vi "HasCommandArray_Query.vi"(0 "System no.":i32=1 min=1 max=4 step=1, 1 "Command":string[](array[string]), 3 "Check HLP?":bool, 4 "HLP? answer":string, 5 "error in":errorcluster) -> (14 "Available GCS commands":string[](array[string]), 15 "Is command available?":bool[](array[boolean]), 19 "error out":errorcluster)   [LabVIEW 2020]
doc: "Polymorphic VI instance for Is command present in HLP? answer.vi.\nThis VI checks whether the specified commands are present in the HLP? answer.\n\nIf Check HLP? is TRUE, HLP?.vi will be called to get HLP? information.\nIf Check HLP? is FALSE, a valid HLP? answer has to be provided in HLP answer."
panel:
  # "Is Command present in HLP answer?.vi\n\nThis VI checks whether the specified commands are present in the HLP? answer.\n\nIf \"Check HLP?\" is TRUE, HLP?.vi will be called to get HLP? information.\nIf \"Check HLP?\" is FALSE, a valid HLP? answer has to be provided in \"HLP answer\"."
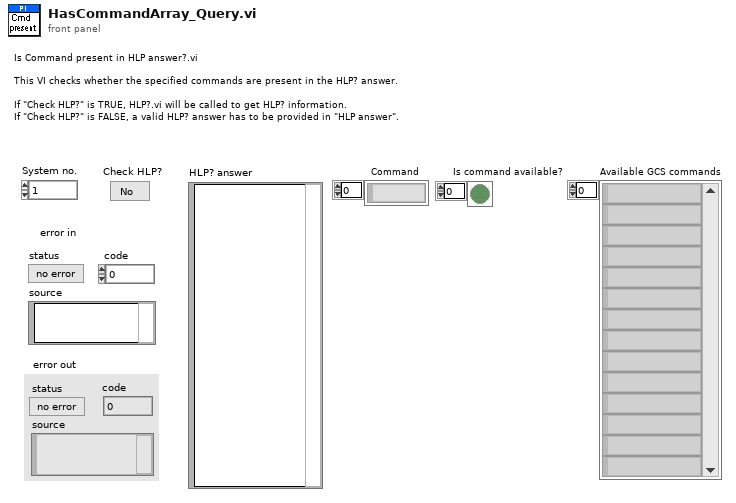
[diagram p1: front panel]
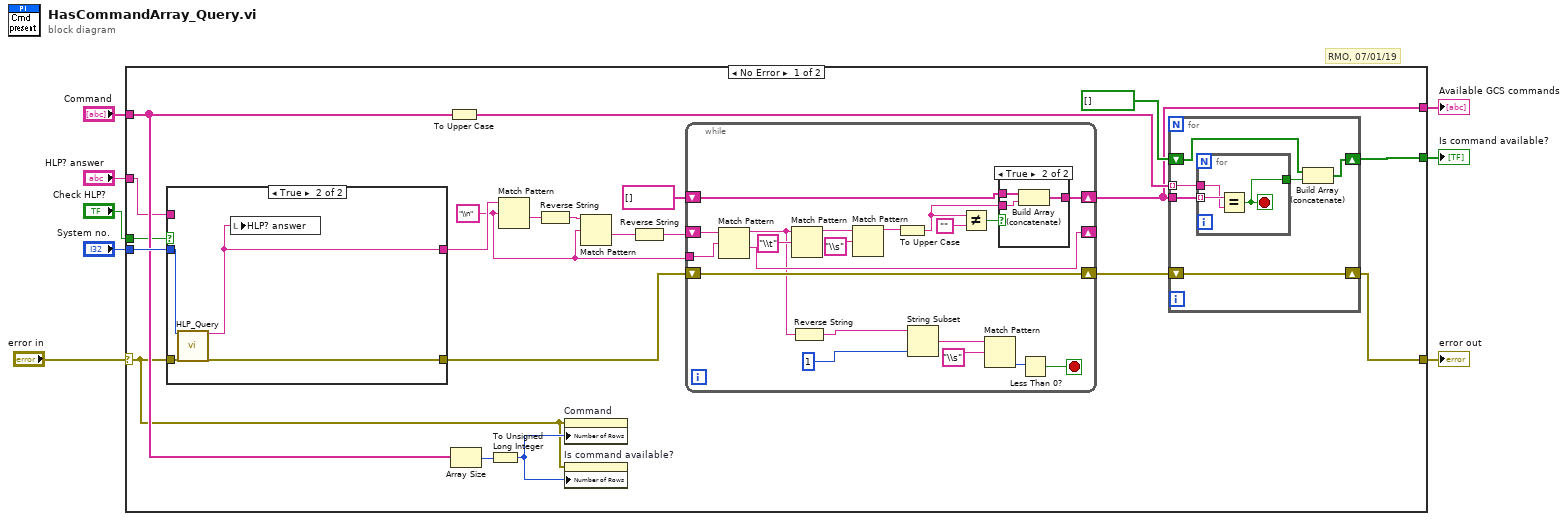
[diagram p0: block diagram]
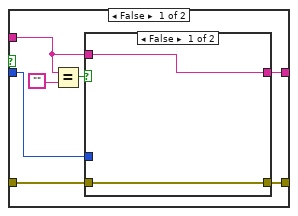
[diagram p2: hidden frame]
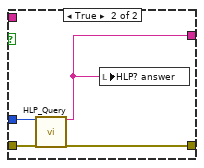
[diagram p3: hidden frame]
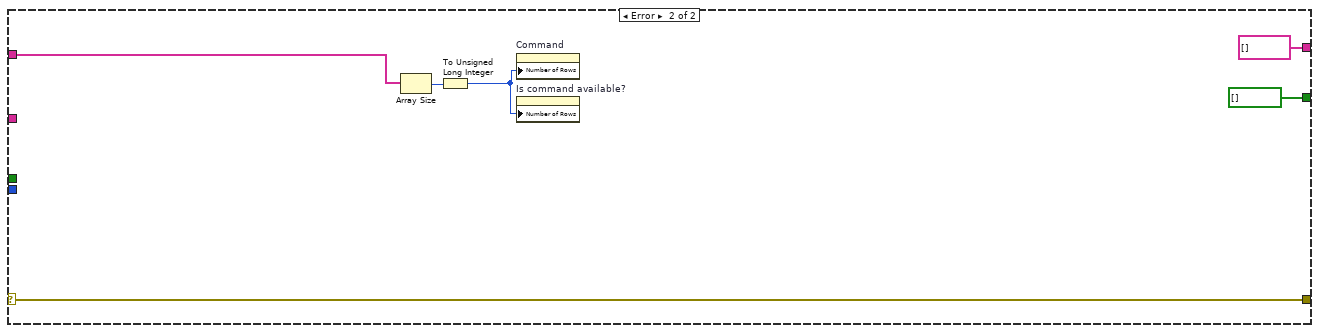
[diagram p5: hidden frame]
diagram:
  # "RMO, 07/01/19"
  n1 = case shown="No Error" "error in" {
    selector: "error in" -> [w9 w80]
    tunnel: [w23 w80] -> w8
    tunnel: "System no." -> [w29 _]
    tunnel: "Command" -> [w14 w82]
    tunnel: [w22 string[] []] -> w5
    tunnel: [w21 bool[] []] -> w4
    tunnel: "Check HLP?" -> [w11 _]
    tunnel: "HLP? answer" -> [w10 _]
    frame No Error {
      w17 = "\\n" ("regular expression")
      n2 = case shown="True" w11 {
        tunnel: w29 -> [w32 w46]
        tunnel: [w30 w43] -> w20
        tunnel: [w33 w45] -> w15
        tunnel: w9 -> [w34 w44]
        tunnel: w10 -> [w31 _]
        frame False {
          n3 = Equal?(x=w31, y="") -> (x = y?=w35:bool)
          n4 = case shown="False" w35 {
            tunnel: w34 -> [w38 w42]
            tunnel: [w38 w41] -> w33
            tunnel: w32 -> [_ w40]
            tunnel: w31 -> [w37 _]
            tunnel: [w37 w39] -> w30
            frame False {
            }
            frame True {
              n5 = call "HLP_Query.vi"("System no."=w40, "error in"=w42) -> ("Help string"=w39:string, "error out"=w41:errorcluster)  [unwired: 16 out]
              n6 = local write "HLP? answer"(w39) -> ()
            }
          }
        }
        frame True {
          n7 = call "HLP_Query.vi"("System no."=w46, "error in"=w44) -> ("Help string"=w43:string, "error out"=w45:errorcluster)  [unwired: 16 out]
          n8 = local write "HLP? answer"(w43) -> ()
        }
      }
      n9 = To Upper Case(1:w14) -> (0:w26:string[])
      n10 = Array Size(array=w14) -> (size(s)=w13:i32)
      n11 = To Unsigned Long Integer(number=w13) -> (unsigned 32bit integer=w12:u32)
      n12 = Match Pattern(string=w20, regular expression=w17) -> (after substring=w19:string)  [unwired: 4 out]
      n13 = Reverse String(1:w19) -> (0:w18:string)
      n14 = property on="Command" class="Arr (strict)"(error in=w9, "Number of Rows"=w12) -> ()  [unwired: 1 in, 2 out]
      n15 = property on="Is command available?" class="Arr (strict)"(error in=w9, "Number of Rows"=w12) -> ()  [unwired: 1 in, 2 out]
      n16 = Match Pattern(string=w18, regular expression=w17) -> (after substring=w16:string)  [unwired: 4 out]
      n17 = Reverse String(1:w16) -> (0:w28:string)
      n18 = while {
        tunnel: w17 -> [w69]
        shift-right: [w65] -> _
        shift-left: w28 -> [w68]
        shift-right: [w73] -> w22
        shift-left: string[] [] -> [w74]
        shift-right: [w67] -> w24
        shift-left: w15 -> [w67]
        stop <- w75 stop-if-true
        n19 = Match Pattern(string=w68, regular expression=w69) -> (before substring=w63:string, after substring=w65:string)  [unwired: 3 out]
        n20 = Match Pattern(string=w63, regular expression="\\t") -> (before substring=w58:string)  [unwired: 4 out]
        n21 = Reverse String(1:w63) -> (0:w62:string)
        n22 = Match Pattern(string=w58, regular expression="\\s") -> (before substring=w56:string)  [unwired: 4 out]
        n23 = To Upper Case(1:w56) -> (0:w72:string)
        n24 = String Subset(string=w62, length (rest)=1) -> (substring=w60:string)  [unwired: 1 out]
        n25 = Not Equal?(x=w72, y="") -> (x != y?=w70:bool)
        n26 = Match Pattern(string=w60, regular expression="\\s") -> (offset past match=w64:i32)  [unwired: 4 out]
        n27 = case shown="True" w70 {
          tunnel: w74 -> [w76 w79]
          tunnel: [w76 w78] -> w73
          tunnel: w72 -> [_ w77]
          frame False {
          }
          frame True {
            n28 = Build Array (concatenate)(w79, w77) -> (w78:string[])
          }
        }
        n29 = Less Than 0?(x=w64) -> (x < 0?=w75:bool)
      }
      n30 = for {
        tunnel: w22 -> [w51]
        tunnel: w26 -> [w52] mode=indexing
        shift-right: [w48] -> w21
        shift-left: bool[] [] -> [w49]
        shift-right: [w47] -> w23
        shift-left: w24 -> [w47]
        n31 = for {
          tunnel: w52 -> [w54]
          tunnel: w51 -> [w55] mode=indexing
          tunnel: [w53] -> w50
          stop <- w53 stop-if-true
          n32 = Equal?(x=w55, y=w54) -> (x = y?=w53:bool)
        }
        n33 = Build Array (concatenate)(w49, w50) -> (w48:bool[])
      }
    }
    frame Error {
      n34 = Array Size(array=w82) -> (size(s)=w83:i32)
      n35 = To Unsigned Long Integer(number=w83) -> (unsigned 32bit integer=w81:u32)
      n36 = property on="Command" class="Arr (strict)"("Number of Rows"=w81) -> ()  [unwired: 2 in, 2 out]
      n37 = property on="Is command available?" class="Arr (strict)"("Number of Rows"=w81) -> ()  [unwired: 2 in, 2 out]
    }
  }
  "error out" <- w8
  "Available GCS commands" <- w5
  "Is command available?" <- w4
